vi "Close Ref.vi"(8 "error in (no error)":errorcluster, 11 "Agilent 3054A in":refnum<class "Agilent 3054A.lvclass">) -> (0 "error out":errorcluster, 3 "Agilent 3054A out":refnum<class "Agilent 3054A.lvclass">)   [LabVIEW 2016, in "Oscilloscope.lvlib" / "Agilent 3054A.lvclass"]
uses:
  Agilent 3054A.lvclass
  Agilent 3054A.lvclass/Agilent 3054A.ctl
  <instrlib>/Agilent 2000 3000 X-Series/Agilent 2000 3000 X-Series.lvlib
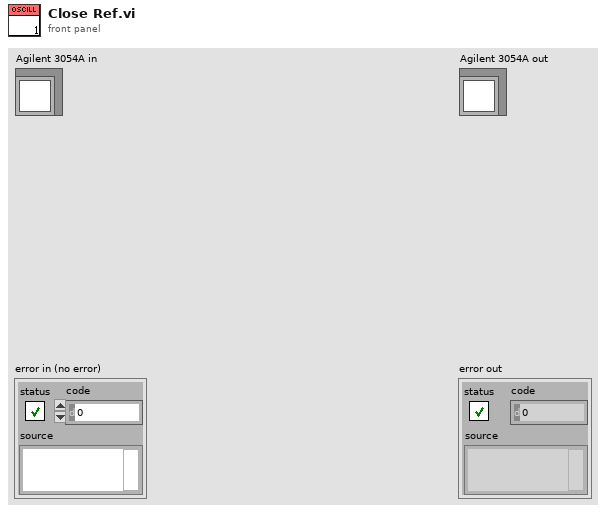
[diagram p1: front panel]
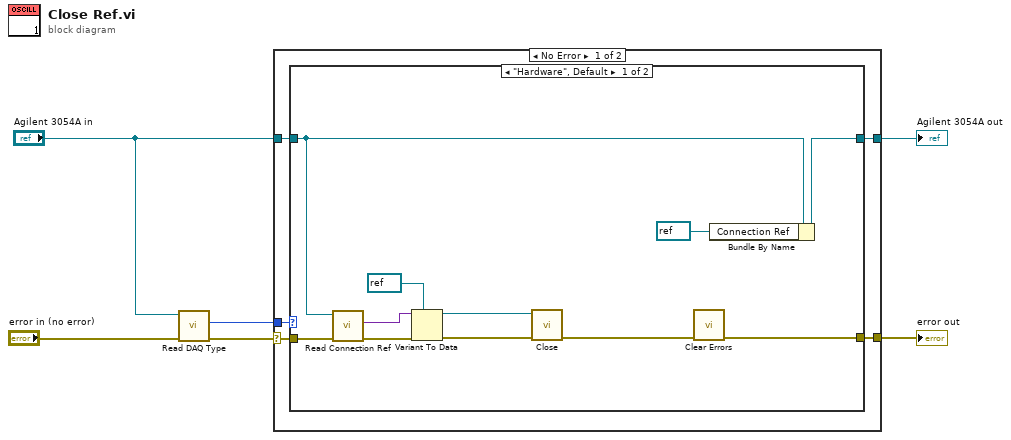
[diagram p0: block diagram]
diagram:
  n1 = call-dynamic "Read DAQ Type.vi"("error in (no error)"="error in (no error)", "Agilent 3054A in"="Agilent 3054A in") -> ("error out"=w5:errorcluster, "DAQ Type"=w4:enum16{"Hardware", "Simulation"})  [unwired: 7 in, 1 out]
  n2 = case shown="No Error" w5 {
    selector: w5 -> [w10 w25]
    tunnel: w4 -> [w11 _]
    tunnel: "Agilent 3054A in" -> [w9 w26]
    tunnel: [w8 w26] -> w2
    tunnel: [w7 w25] -> w1
    frame No Error {
      n3 = case shown="\"Hardware\", Default" w11 {
        tunnel: w10 -> [w22 w23]
        tunnel: w9 -> [w16 w24]
        tunnel: [w14 w24] -> w8
        tunnel: [w12 w23] -> w7
        frame "Hardware", Default {
          n4 = call-dynamic "Read Connection Ref.vi"("error in (no error)"=w22, "Agilent 3054A in"=w16) -> ("error out"=w21:errorcluster, "Connection Ref"=w19:variant)  [unwired: 7 in, 1 out]
          n5 = Variant To Data(error in=w21, type=refnum<visa-resource-name> refnum ("VISA resource name"), Variant=w19) -> (data=w18:refnum<visa-resource-name>, error out=w17:errorcluster)
          n6 = call <instrlib>:"Close.vi"("error in (no error)"=w17, "VISA resource name"=w18) -> ("error out"=w15:errorcluster)  [unwired: 9 in]
          n7 = call <vilib>:"Clear Errors.vi"("error in (no error)"=w15) -> ("error out"=w12:errorcluster)  [unwired: 5 in, 1 out]
          n8 = Bundle By Name(cluster=w16, "Connection Ref"=refnum<visa-resource-name> refnum ("VISA resource name")) -> (w14:refnum<class "Agilent 3054A.lvclass">)
        }
        frame "Simulation" {
        }
      }
    }
    frame Error {
    }
  }
  "error out" <- w1
  "Agilent 3054A out" <- w2
